vi "testNoMeasured.vi"() -> ()   [LabVIEW 2017, in "CodeCoverageTest.lvlib"]
uses:
  CodeCoverageTest.lvlib
  CodeCoverage/CodeCoverage.lvclass
  Assertion/Assertion.lvlib
panel:
  out "error out":errorcluster
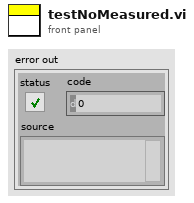
[diagram p1: front panel]
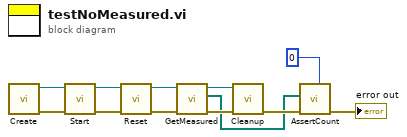
[diagram p0: block diagram]
diagram:
  n1 = call "Create.vi"() -> ("error out"=w11:errorcluster, "CodeCoverage out"=w12:refnum<class "CodeCoverage.lvclass">)  [unwired: 10 in]
  n2 = call "Start.vi"("error in (no error)"=w11, "CodeCoverage in"=w12) -> ("error out"=w9:errorcluster, "CodeCoverage out"=w10:refnum<class "CodeCoverage.lvclass">)  [unwired: 8 in]
  n3 = call "Reset.vi"("error in (no error)"=w9, "CodeCoverage in"=w10) -> ("error out"=w7:errorcluster, "CodeCoverage out"=w8:refnum<class "CodeCoverage.lvclass">)  [unwired: 8 in]
  n4 = call "GetMeasured.vi"("error in (no error)"=w7, "CodeCoverage in"=w8) -> ("error out"=w5:errorcluster, "All VIs Measured"=w3:path[], "CodeCoverage out"=w6:refnum<class "CodeCoverage.lvclass">)  [unwired: 7 in]
  n5 = call "Cleanup.vi"("error in (no error)"=w5, "CodeCoverage in"=w6) -> ("error out"=w4:errorcluster)  [unwired: 9 in]
  n6 = call "AssertCount.vi"("Expected"=0, "error in (no error)"=w4, "Haystack"=w3) -> ("error out"=→"error out":errorcluster)  [unwired: 8 in]
